vi "Init Logger.vi"(8 "error in (no error)":errorcluster, 10 "File Send Interval (Seconds)":dbl=600.0) -> (0 "error out":errorcluster, 3 "Logger out.lvclass":refnum<class "Logger.lvclass">)   [LabVIEW 2018, in "Logger.lvclass"]
uses:
  Logger.lvclass
  <vilib>/Skyline/Tag/Wrapper/Wrapper_class/Tag Value Cluster Wrapper.ctl
  <vilib>/Skyline/Configuration/Configuration_class/NI Skyline Configuration.lvclass
  <vilib>/Skyline/Tag/Shared/typedefs/Tag Value Cluster.ctl
  <vilib>/Skyline/Tag/Shared/typedefs/DataType.ctl
  <vilib>/Skyline/Tag/Wrapper/Wrapper_class/NI Skyline Tag.lvclass
  <vilib>/Skyline/Tag/Shared/typedefs/TagProperty.ctl
  Logger.lvclass/Logger.ctl
  <vilib>/Skyline/Tag/Wrapper/Wrapper AMQP_class/Open Tag AMQP.vi
  <vilib>/Skyline/Tag/Wrapper/Wrapper_class/Generate Tag Cluster (String) 2.vi
  <vilib>/Skyline/Tag/Wrapper/Wrapper_class/Generate Tag Cluster (I32) 2.vi
  <vilib>/Skyline/Message/AMQP/sync/Open (Sync).vi
  <vilib>/Skyline/Message/AMQP/NI Skyline Message AMQP (Sync).lvclass
  <vilib>/Skyline/Tag/Shared/NI Skyline Tag.lvlib
  <vilib>/Skyline/Tag/Wrapper/Wrapper AMQP_class/NI Skyline Tag AMQP.lvclass
  <vilib>/Skyline/Message/NI Skyline Message.lvclass
  <vilib>/Skyline/Utilities/NI Skyline Utilities.lvlib
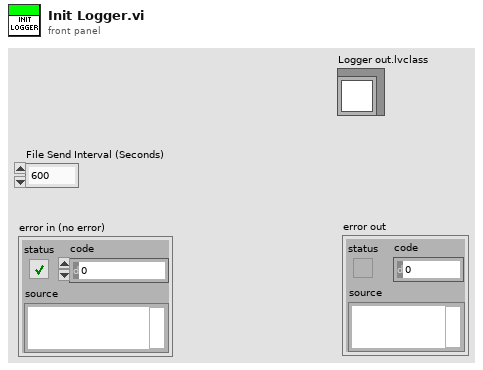
[diagram p1: front panel]
types:
  T1 = typedef "NI Skyline Tag.lvclass/Tag Value Cluster Wrapper.ctl" = cluster{"Configuration":refnum<class "NI Skyline Configuration.lvclass">, "Tag Cluster":T2}
  T2 = typedef "NI Skyline Tag.lvlib/Tag Value Cluster.ctl" = cluster{"Path":string, "Data Type":T3, "Value":string, "Time Stamp":timestamp}
  T3 = typedef "NI Skyline Tag.lvlib/DataType.ctl" = enum32{"Double", "I32", "String", "Boolean", "U64", "Timestamp"}
  T4 = typedef "NI Skyline Tag.lvlib/TagProperty.ctl" = cluster{"key":string, "value":string}
  T5 = cluster{"Tag Units":string, "Tag Path":string, "Waveform":waveform(dbl), "Log":bool, "Tag Reference":refnum<class "NI Skyline Tag.lvclass">}
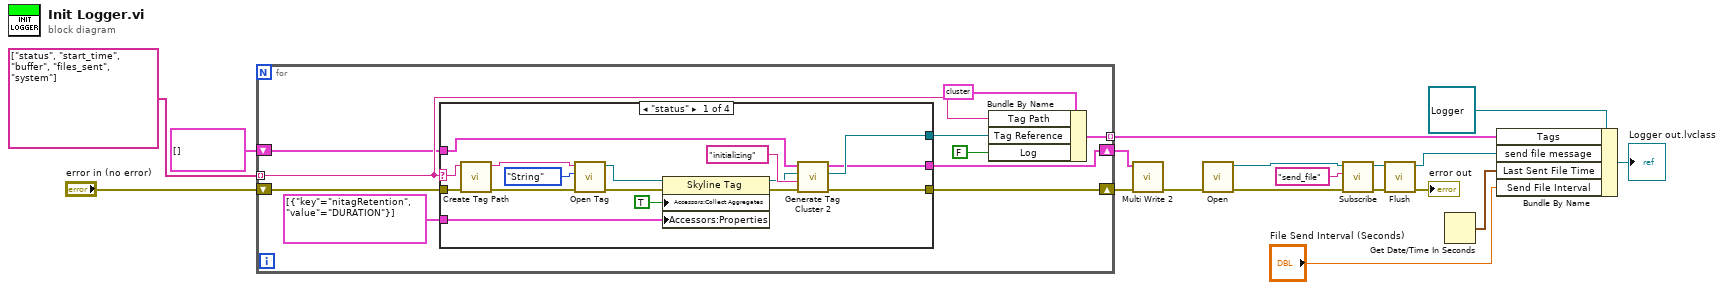
[diagram p0: block diagram]
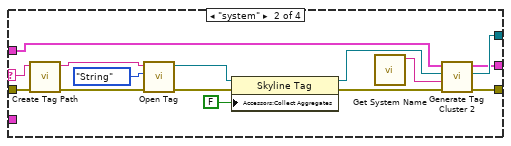
[diagram p2: hidden frame]
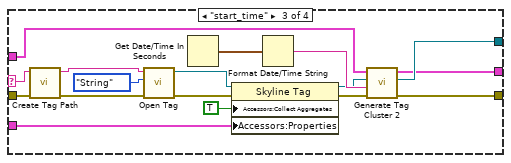
[diagram p3: hidden frame]
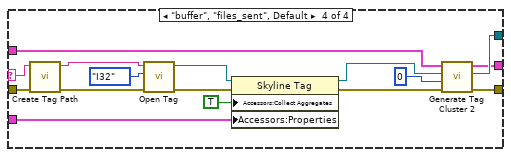
[diagram p4: hidden frame]
diagram:
  n1 = for {
    shift-right: [w28] -> w13
    shift-left: "error in (no error)" -> [w25]
    tunnel: string[] ["status", "start_time", "buffer", "files_sent", "system"] -> [w26] mode=indexing
    tunnel: [w27] -> w11 mode=indexing
    shift-right: [w21] -> w7
    shift-left: T1[] [] ("tag clusters out") -> [w22]
    n2 = case shown="\"status\"" w26 {
      selector: w26 -> [w43 w58 w61 w82]
      tunnel: [w41 w56 w73 w91] -> w28
      tunnel: [w42 w57 w74 w92] -> w23
      tunnel: w25 -> [w44 w59 w62 w81]
      tunnel: [w37 w52 w71 w89] -> w21
      tunnel: w22 -> [w30 w46 w72 w88]
      tunnel: T4[] [{"key"="nitagRetention", "value"="DURATION"}] ("Properties") -> [w29 _ w60 w77]
      frame "status" {
        n3 = call "Create Tag Path.vi"("error in (no error)"=w44, "tag name"=w43) -> ("error out"=w40:errorcluster, "path"=w39:string)  [unwired: 8 in]
        n4 = call-poly <vilib>:"Open Tag.vi"("error in (no error)"=w40, "data type"=DataType."String" ("Data Type"), "path"=w39) -> ("error out"=w33:errorcluster, "tag out"=w34:refnum<class "NI Skyline Tag.lvclass">)  [unwired: 7 in]
        n5 = property on="Property Node" class="Skyline Tag"(reference=w34, error in=w33, "Accessors:Collect Aggregates"=TRUE ("Collect Aggregates"), "Accessors:Properties"=w29) -> (reference out=w32:refnum<class "NI Skyline Tag.lvclass">, error out=w31:errorcluster)
        n6 = call-poly <vilib>:"Generate Tag Cluster 2.vi"("error in (no error)"=w31, "value"="initializing" ("string"), "tag in"=w32, "tag clusters in"=w30) -> ("error out"=w41:errorcluster, "tag out"=w42:refnum<class "NI Skyline Tag.lvclass">, "tag clusters out"=w37:T1[])  [unwired: 5 in]
      }
      frame "system" {
        n7 = call "Create Tag Path.vi"("error in (no error)"=w59, "tag name"=w58) -> ("error out"=w55:errorcluster, "path"=w54:string)  [unwired: 8 in]
        n8 = call-poly <vilib>:"Open Tag.vi"("error in (no error)"=w55, "data type"=DataType."String" ("Data Type"), "path"=w54) -> ("error out"=w49:errorcluster, "tag out"=w50:refnum<class "NI Skyline Tag.lvclass">)  [unwired: 7 in]
        n9 = property on="Property Node" class="Skyline Tag"(reference=w50, error in=w49, "Accessors:Collect Aggregates"=FALSE ("Collect Aggregates")) -> (reference out=w48:refnum<class "NI Skyline Tag.lvclass">, error out=w47:errorcluster)
        n10 = call <vilib>:"Get System Name.vi"() -> ("system name"=w45:string)  [unwired: 11 in]
        n11 = call-poly <vilib>:"Generate Tag Cluster 2.vi"("error in (no error)"=w47, "value"=w45, "tag in"=w48, "tag clusters in"=w46) -> ("error out"=w56:errorcluster, "tag out"=w57:refnum<class "NI Skyline Tag.lvclass">, "tag clusters out"=w52:T1[])  [unwired: 5 in]
      }
      frame "start_time" {
        n12 = call "Create Tag Path.vi"("error in (no error)"=w62, "tag name"=w61) -> ("error out"=w63:errorcluster, "path"=w64:string)  [unwired: 8 in]
        n13 = call-poly <vilib>:"Open Tag.vi"("error in (no error)"=w63, "data type"=DataType."String" ("Data Type"), "path"=w64) -> ("error out"=w67:errorcluster, "tag out"=w68:refnum<class "NI Skyline Tag.lvclass">)  [unwired: 7 in]
        n14 = Get Date/Time In Seconds() -> (seconds since 1Jan1904=w76:timestamp)
        n15 = property on="Property Node" class="Skyline Tag"(reference=w68, error in=w67, "Accessors:Collect Aggregates"=TRUE ("Collect Aggregates"), "Accessors:Properties"=w60) -> (reference out=w66:refnum<class "NI Skyline Tag.lvclass">, error out=w65:errorcluster)
        n16 = Format Date/Time String(seconds (now)=w76) -> (date/time string=w70:string)  [unwired: 2 in]
        n17 = call-poly <vilib>:"Generate Tag Cluster 2.vi"("error in (no error)"=w65, "value"=w70, "tag in"=w66, "tag clusters in"=w72) -> ("error out"=w73:errorcluster, "tag out"=w74:refnum<class "NI Skyline Tag.lvclass">, "tag clusters out"=w71:T1[])  [unwired: 5 in]
      }
      frame "buffer", "files_sent", Default {
        n18 = call "Create Tag Path.vi"("error in (no error)"=w81, "tag name"=w82) -> ("error out"=w80:errorcluster, "path"=w79:string)  [unwired: 8 in]
        n19 = call-poly <vilib>:"Open Tag.vi"("error in (no error)"=w80, "data type"=DataType."I32", "path"=w79) -> ("error out"=w86:errorcluster, "tag out"=w87:refnum<class "NI Skyline Tag.lvclass">)  [unwired: 7 in]
        n20 = property on="Property Node" class="Skyline Tag"(reference=w87, error in=w86, "Accessors:Collect Aggregates"=TRUE ("Collect Aggregates"), "Accessors:Properties"=w77) -> (reference out=w84:refnum<class "NI Skyline Tag.lvclass">, error out=w83:errorcluster)
        n21 = call-poly <vilib>:"Generate Tag Cluster 2.vi"("error in (no error)"=w83, "value"=0, "tag in"=w84, "tag clusters in"=w88) -> ("error out"=w91:errorcluster, "tag out"=w92:refnum<class "NI Skyline Tag.lvclass">, "tag clusters out"=w89:T1[])  [unwired: 5 in]
      }
    }
    n22 = Bundle By Name(cluster=T5 {"Tag Units"="", "Tag Path"="", "Waveform"={"t0"=timestamp(0 s since 1904-01-01), "dt"=1.0, "Y"=[]}, "Log"=FALSE, "Tag Reference"=refnum} ("Tag"), "Tag Path"=w26, "Tag Reference"=w23, "Log"=FALSE) -> (w27:T5)
  }
  n23 = call <vilib>:"Multi Write 2.vi"("error in (no error)"=w13, "tag clusters"=w7) -> ("error out"=w12:errorcluster)  [unwired: 9 in]
  n24 = call-poly <vilib>:"Open.vi"("error in (no error)"=w12) -> ("error out"=w4:errorcluster, "message sync out"=w5:refnum<class "NI Skyline Message AMQP (Sync).lvclass">)  [unwired: 9 in]
  n25 = call-dynamic "Subscribe.vi"("error in (no error)"=w4, "topic"="send_file" ("Tag"), "message sync"=w5) -> ("error out"=w3:errorcluster, "message sync out"=w2:refnum<class "NI Skyline Message AMQP (Sync).lvclass">)  [unwired: 7 in]
  n26 = call-dynamic "Flush.vi"("error in (no error)"=w3, "message sync"=w2) -> ("error out"=→"error out":errorcluster, "message sync out"=w10:refnum<class "NI Skyline Message AMQP (Sync).lvclass">)  [unwired: 8 in]
  n27 = Get Date/Time In Seconds() -> (seconds since 1Jan1904=w16:timestamp)
  n28 = Bundle By Name(cluster=refnum<class "Logger.lvclass"> refnum ("Logger out.lvclass"), "Tags"=w11, "send file message"=w10, "Last Sent File Time"=w16, "Send File Interval"="File Send Interval (Seconds)") -> (→"Logger out.lvclass":refnum<class "Logger.lvclass">)
